vi "Check Axes Compatibility of Named Positions.vi"(10 "Num Axes":i32, 11 "named_position":T1) -> (0 "error out":errorcluster, 3 "named_position":T1)   [LabVIEW 2020, in "Manipulator.lvlib"]
uses:
  Manipulator.lvlib
  Settings/Named Position.ctl
  <vilib>/Utility/error.llb/Error Cluster From Error Code.vi
  <vilib>/ErrorRing/Error Ring.xnode
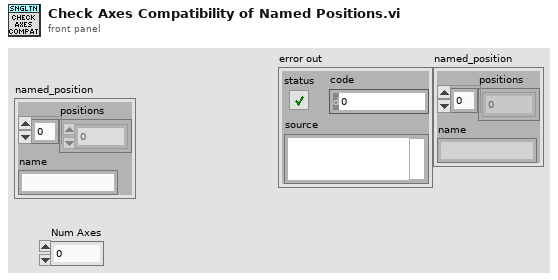
[diagram p1: front panel]
types:
  T1 = typedef "Manipulator.lvlib/Named Position.ctl" = cluster{"positions":dbl[], "name":string}
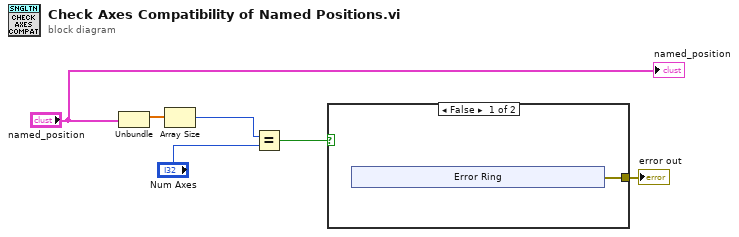
[diagram p0: block diagram]
diagram:
  n1 = Unbundle("named_position") -> ("positions"=w5:dbl[])  [unwired: 1 out]
  n2 = Array Size(array=w5) -> (size(s)=w4:i32)
  n3 = Equal?(x=w4, y="Num Axes") -> (x = y?=w2:bool)
  n4 = case shown="False" w2 {
    tunnel: [w7 _] -> w1
    frame False {
      n5 = xnode "Error Ring"() -> ("error out"=w7:errorcluster)
    }
    frame True {
    }
  }
  "error out" <- w1
  "named_position" <- "named_position"
